vi "test_AfterCallUnreserveSessions_SessionReservationReturnsErrorForAnyAction.vi"(8 "error in":errorcluster) -> (0 "error out":errorcluster, 2 "result":string, 3 "pass":bool)   [LabVIEW 2020, in "MeasurementServerTests.lvlib"]
uses:
  Helpers/Fake Instrument/Fake Instrument.lvclass
  \\tsclient\C/dev/measurementlink-labview/Source/Runtime/MeasurementLink Instrument/IInstrument/IInstrument.lvclass
  Runtime/MeasurementLink Measurement Server/Helpers/Error Strings Global Internal.vi
  Runtime/MeasurementLink Session Management/Session Reservation/Create Sessions Impl.vi
  MeasurementServerTests.lvlib
  da6ffb6f-c1c9-4957-84dd-e9228483c454.vi
  Runtime/MeasurementLink Session Management/Session Reservation/Session Reservation.lvclass
  4bbddc2a-be03-47e4-8644-5d4b5205751b.vi
  34973808-273d-4b1e-ac93-8b9a23c2e7c8.vi
  b8e3467f-0abf-4dd6-b6da-3b4f4c560b3c.vi
  44116b28-3318-4200-87c4-820acb1f6e49.vi
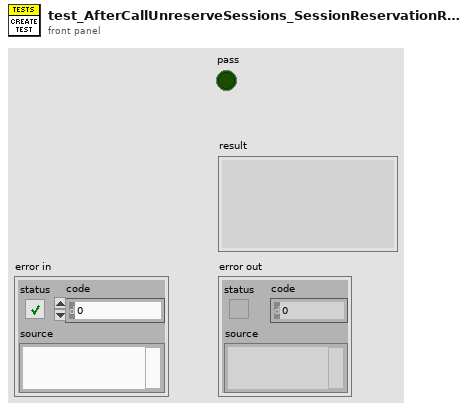
[diagram p1: front panel]
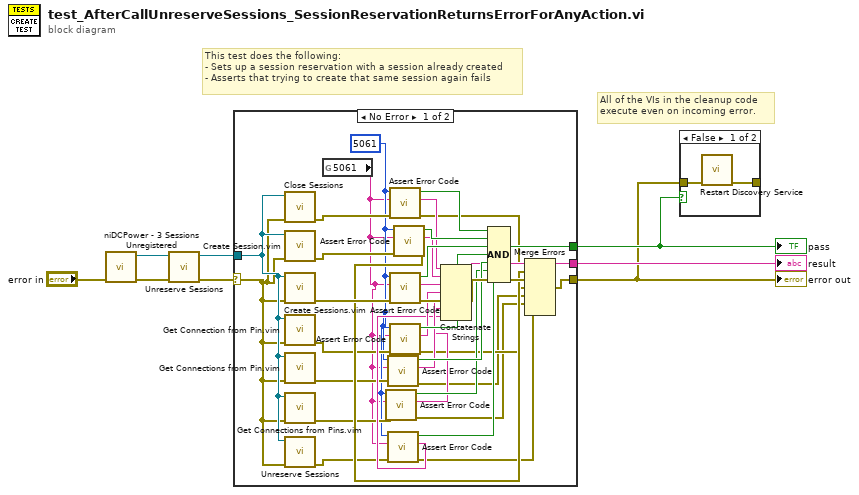
[diagram p0: block diagram]
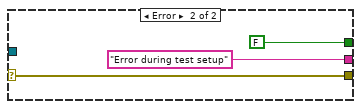
[diagram p2: hidden frame]
diagram:
  # "All of the VIs in the cleanup code\nexecute even on incoming error."
  # "This test does the following:\n- Sets up a session reservation with a session already created\n- Asserts that trying to create that same session again fails"
  n1 = call "niDCPower - 3 Sessions Unregistered.vi"("error in (no error)"="error in") -> ("error out"=w3:errorcluster, "Session Reservation out"=w2:refnum<class "Session Reservation.lvclass">)  [unwired: 9 in]
  n2 = call "Unreserve Sessions.vi"("error in"=w3, "session reservation in"=w2) -> ("error out"=w5:errorcluster, "session reservation out"=w1:refnum<class "Session Reservation.lvclass">)  [unwired: 8 in]
  n3 = case shown="No Error" w5 {
    selector: w5 -> [w9 w44]
    tunnel: [w25 w44] -> w6
    tunnel: [w39 FALSE] -> w7
    tunnel: [w32 "Error during test setup" ("f")] -> w8
    tunnel: w1 -> [w10 _]
    frame No Error {
      w12 = 5061 ("expected error code")
      n4 = call "Close Sessions.vi"("error in"=w9, "session reservation in"=w10) -> ("error out"=w18:errorcluster)  [unwired: 8 in, 1 out]
      n5 = call "Create Session.vim"("error in"=w9, "session reservation in"=w10) -> ("error out"=w17:errorcluster)  [unwired: 6 in, 3 out]
      n6 = call "Create Sessions.vim"("error in"=w9, "session reservation in"=w10) -> ("error out"=w43:errorcluster)  [unwired: 6 in, 3 out]
      n7 = call "Get Connection from Pin.vim"("error in"=w9, "session reservation in"=w10) -> ("error out"=w16:errorcluster)  [unwired: 7 in, 2 out]
      n8 = call "Get Connections from Pin.vim"("error in"=w9, "session reservation in"=w10) -> ("error out"=w15:errorcluster)  [unwired: 7 in, 2 out]
      n9 = call "Get Connections from Pins.vim"("error in"=w9, "session reservation in"=w10) -> ("error out"=w14:errorcluster)  [unwired: 7 in, 2 out]
      n10 = call "Unreserve Sessions.vi"("error in"=w9, "session reservation in"=w10) -> ("error out"=w13:errorcluster)  [unwired: 8 in, 1 out]
      n11 = global read "Error Strings Global Internal.vi" "5061"() -> (w11:string)
      n12 = call "Assert Error Code.vi"("error in"=w14, "expected error description"=w11, "expected error code"=w12) -> ("error out"=w20:errorcluster, "details"=w27:string, "error code match?"=w36:bool)  [unwired: 6 in]
      n13 = call "Assert Error Code.vi"("error in"=w15, "expected error description"=w11, "expected error code"=w12) -> ("error out"=w21:errorcluster, "details"=w28:string, "error code match?"=w37:bool)  [unwired: 6 in]
      n14 = call "Assert Error Code.vi"("error in"=w13, "expected error description"=w11, "expected error code"=w12) -> ("error out"=w19:errorcluster, "details"=w26:string, "error code match?"=w35:bool)  [unwired: 6 in]
      n15 = call "Assert Error Code.vi"("error in"=w18, "expected error description"=w11, "expected error code"=w12) -> ("error out"=w24:errorcluster, "details"=w31:string, "error code match?"=w33:bool)  [unwired: 6 in]
      n16 = call "Assert Error Code.vi"("error in"=w43, "expected error description"=w11, "expected error code"=w12) -> ("error out"=w41:errorcluster, "details"=w40:string, "error code match?"=w42:bool)  [unwired: 6 in]
      n17 = call "Assert Error Code.vi"("error in"=w16, "expected error description"=w11, "expected error code"=w12) -> ("error out"=w22:errorcluster, "details"=w29:string, "error code match?"=w38:bool)  [unwired: 6 in]
      n18 = call "Assert Error Code.vi"("error in"=w17, "expected error description"=w11, "expected error code"=w12) -> ("error out"=w23:errorcluster, "details"=w30:string, "error code match?"=w34:bool)  [unwired: 6 in]
      n19 = Concatenate Strings(w31, w30, w40, w29, w28, w27, w26) -> (w32:string)
      n20 = Compound Arithmetic op=AND(w33, w34, w42, w38, w37, w36, w35) -> (w39:bool)
      n21 = Merge Errors(w24, w23, w41, w22, w21, w20, w19) -> (w25:errorcluster)
    }
    frame Error {
    }
  }
  "error out" <- w6
  "pass" <- w7
  "result" <- w8
  n22 = case shown="False" w7 {
    tunnel: w6 -> [w48 _]
    tunnel: [w47 _] -> _
    frame False {
      n23 = call "Restart Discovery Service.vi"("error in"=w48) -> ("error out"=w47:errorcluster)  [unwired: 10 in]
    }
    frame True {
    }
  }
